vi "Read Section Path.vi"(7 "Section Name":string, 8 "error in (no error)":errorcluster, 10 "Section (Cluster)":variant, 11 "Path in":path) -> (0 "error out":errorcluster, 1 "Missing key(s)":bool, 2 "Section (Cluster) out":variant, 3 "Path out":path, 4 "Keys not found":string)   [LabVIEW 2024, in "Generic Config Handling.lvlib"]
doc: "This vi reads the cluster from a section in the config file. \n\nIf section name is not wired then the default is to use the name of the cluster.\n\nEach element of the cluster becomes a key, therefore it must be named, and they should be unique and not include any special characters (spaces are allowed and are replaced by_)\n\nYou cannot nest clusters and only simple datatypes are allowed. 1D and 2D arrays are allowed. They are stored as a single element with columns delimited by semicolons and rows delimited by commas. 1D arrays are stored as a single row (ie. comma delimited). \n\nEnums are stored as U32s.\n\nThe cluster wired to Section is used as the default values for the keys if they are not found. If any key is missing, missing keys is true and a list of missing keys is provided."
uses:
  Generic Config Handling.lvlib
  <vilib>/Utility/config.llb/NI_LVConfig.lvlib
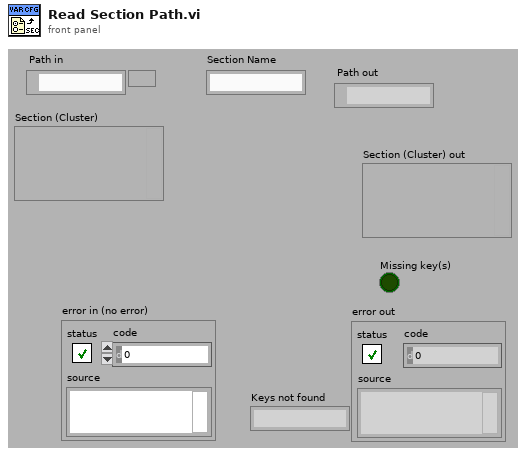
[diagram p1: front panel]
types:
  T1 = typedef "NI_LVConfig.lvlib/Config Data RefNum.ctl" = refnum<k1>
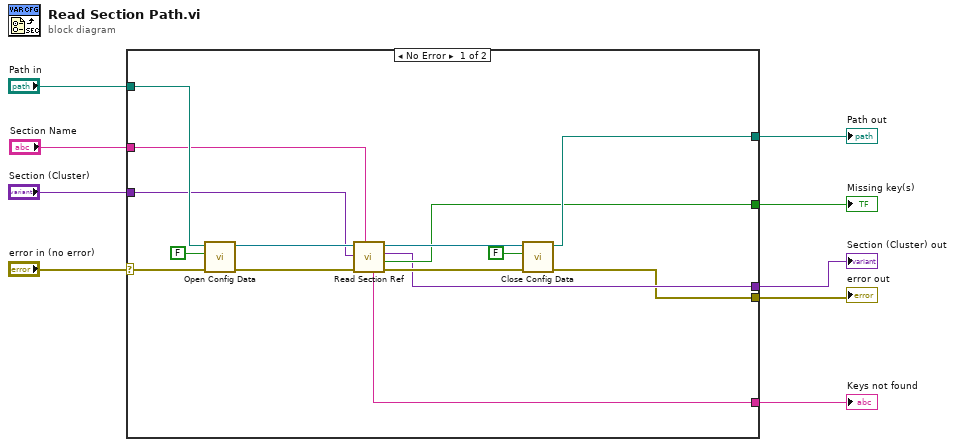
[diagram p0: block diagram]
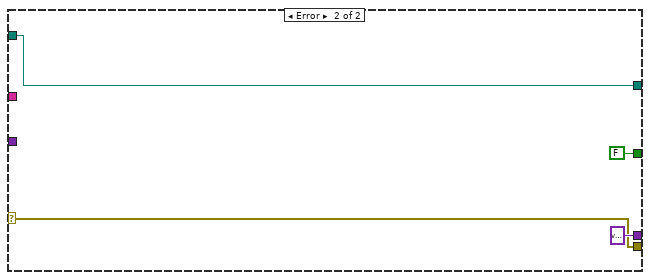
[diagram p2: hidden frame]
diagram:
  n1 = case shown="No Error" "error in (no error)" {
    selector: "error in (no error)" -> [w10 w25]
    tunnel: "Path in" -> [w24 w28]
    tunnel: "Section (Cluster)" -> [w19 _]
    tunnel: "Section Name" -> [w18 _]
    tunnel: [w17 w28] -> w6
    tunnel: [w16 _] -> w5
    tunnel: [w15 FALSE ("Missing key(s)")] -> w4
    tunnel: [w14 variant ("Section (Cluster) out")] -> w3
    tunnel: [w13 w25] -> w2
    frame No Error {
      n2 = call <vilib>:"Open Config Data.vi"("error in (no error)"=w10, "create file if necessary (T)"=FALSE, "configuration file path"=w24) -> ("error out"=w21:errorcluster, "refnum"=w23:T1)  [unwired: 6 in, 1 out]
      n3 = call "Read Section Ref.vi"("Section Name"=w18, "error in (no error)"=w21, "Section (Cluster)"=w19, "Refnum in"=w23) -> ("error out"=w20:errorcluster, "Missing key(s)"=w15:bool, "Section (Cluster) out"=w14:variant, "Refnum out"=w22:T1, "Keys not found"=w16:string)  [unwired: 3 in]
      n4 = call <vilib>:"Close Config Data.vi"("error in (no error)"=w20, "write file if changed (T)"=FALSE, "refnum"=w22) -> ("error out"=w13:errorcluster, "file path"=w17:path)  [unwired: 7 in]
    }
    frame Error {
    }
  }
  "Path out" <- w6
  "error out" <- w2
  "Section (Cluster) out" <- w3
  "Keys not found" <- w5
  "Missing key(s)" <- w4
